vi "Convert Data to message.vi"(8 "entrée d'erreur (pas d'erreur)":errorcluster, 10 "data":variant) -> (0 "sortie d'erreur":errorcluster, 3 "output cluster message":T1)   [LabVIEW 2018, in "Control-Server.lvclass"]
uses:
  Control/Control-Server/Control-Server.lvclass
  dependecies/ControlsVIs/Clusters-def/Standard Command.ctl
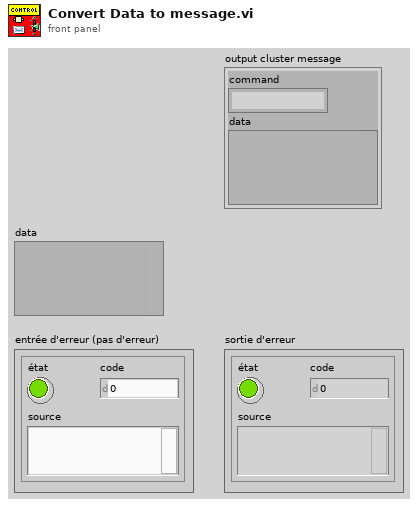
[diagram p1: front panel]
types:
  T1 = typedef "Standard Command.ctl" = cluster{"command":string, "data":variant}
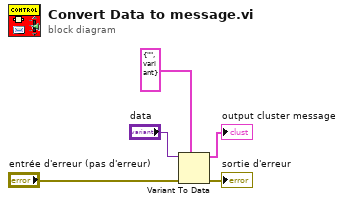
[diagram p0: block diagram]
diagram:
  n1 = Variant To Data(error in="entrée d'erreur (pas d'erreur)", type=T1 {"command"="", "data"=variant} ("input cluster"), Variant="data") -> (data=→"output cluster message":T1, error out=→"sortie d'erreur":errorcluster)
